vi "Auto String Decoder.vi"(8 "Index":i32, 11 "subarray":string[](array[string])) -> (4 "Done with Auto":bool)   [LabVIEW 2017]
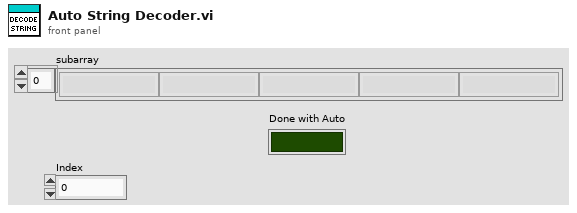
[diagram p1: front panel]
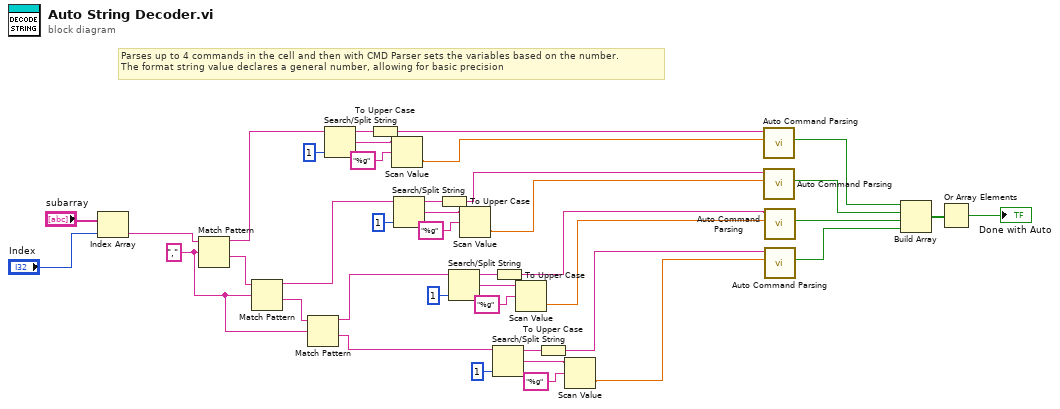
[diagram p0: block diagram]
diagram:
  w34 = "," ("regular expression")
  # "Parses up to 4 commands in the cell and then with CMD Parser sets the variables based on the number.\nThe format string value declares a general number, allowing for basic precision"
  n1 = Index Array(array="subarray", index="Index") -> (element=w23:string)
  n2 = Match Pattern(string=w23, regular expression=w34) -> (before substring=w27:string, after substring=w36:string)  [unwired: 1 in, 2 out]
  n3 = Match Pattern(string=w36, regular expression=w34) -> (before substring=w26:string, after substring=w35:string)  [unwired: 1 in, 2 out]
  n4 = Match Pattern(string=w35, regular expression=w34) -> (before substring=w25:string, after substring=w24:string)  [unwired: 1 in, 2 out]
  n5 = Search/Split String(string=w27, offset (0)=1) -> (substring before match=w38:string, match + rest of string=w2:string)  [unwired: 1 in, 1 out]
  n6 = To Upper Case(1:w38) -> (0:w16:string)
  n7 = Scan Value(string=w2, format string="%g") -> (value=w1:dbl)  [unwired: 1 in, 1 out]
  n8 = Search/Split String(string=w26, offset (0)=1) -> (substring before match=w33:string, match + rest of string=w5:string)  [unwired: 1 in, 1 out]
  n9 = To Upper Case(1:w33) -> (0:w15:string)
  n10 = Search/Split String(string=w25, offset (0)=1) -> (substring before match=w31:string, match + rest of string=w8:string)  [unwired: 1 in, 1 out]
  n11 = Scan Value(string=w5, format string="%g") -> (value=w4:dbl)  [unwired: 1 in, 1 out]
  n12 = Search/Split String(string=w24, offset (0)=1) -> (substring before match=w29:string, match + rest of string=w11:string)  [unwired: 1 in, 1 out]
  n13 = To Upper Case(1:w31) -> (0:w14:string)
  n14 = Scan Value(string=w8, format string="%g") -> (value=w7:dbl)  [unwired: 1 in, 1 out]
  n15 = To Upper Case(1:w29) -> (0:w13:string)
  n16 = Scan Value(string=w11, format string="%g") -> (value=w10:dbl)  [unwired: 1 in, 1 out]
  n17 = call "Auto Command Parsing.vi"("Command Paremeters"=w1, "Command code In"=w16) -> ("Abort"=w20:bool)  [unwired: 8 in, 1 out]
  n18 = call "Auto Command Parsing.vi"("Command Paremeters"=w4, "Command code In"=w15) -> ("Abort"=w19:bool)  [unwired: 8 in, 1 out]
  n19 = call "Auto Command Parsing.vi"("Command Paremeters"=w7, "Command code In"=w14) -> ("Abort"=w18:bool)  [unwired: 8 in, 1 out]
  n20 = call "Auto Command Parsing.vi"("Command Paremeters"=w10, "Command code In"=w13) -> ("Abort"=w17:bool)  [unwired: 8 in, 1 out]
  n21 = Build Array(w20, w19, w18, w17) -> (w22:bool[])
  n22 = Or Array Elements(Boolean array=w22) -> (logical OR=→"Done with Auto":bool)
